vi "stop.vi"(3 "error in (no error)":errorcluster, 4 "stop":bool, 5 "A66xxSupply in":refnum<class "A66xxSupply.lvclass">) -> (0 "error out":errorcluster, 1 "Stopped":bool, 2 "A66xxSupply out":refnum<class "A66xxSupply.lvclass">)   [LabVIEW 2011, in "Hardware.lvlib" / "Channels.lvlib" / "A66xxSupply.lvclass"]
doc: "Abstract Method.\n\nStops the analog output. This vi indicates of the analog output has stopped, and can be used to actively stop the output."
uses:
  A66xxSupply.lvclass
  AnalogOutput.lvclass
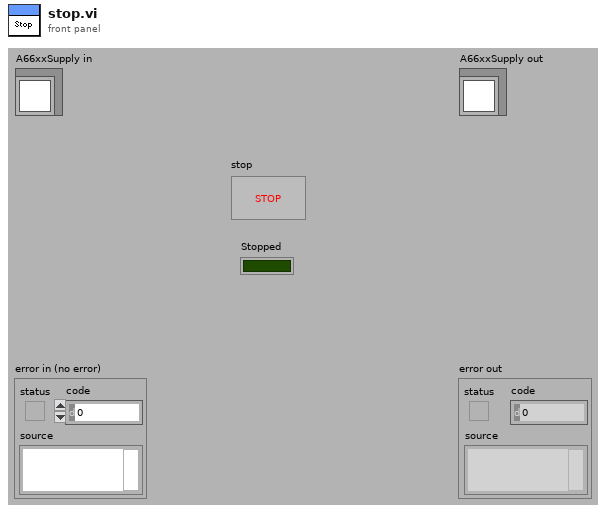
[diagram p1: front panel]
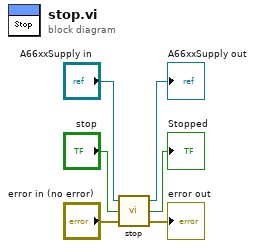
[diagram p0: block diagram]
diagram:
  n1 = call-parent "stop.vi"("error in (no error)"="error in (no error)", "stop"="stop", "AnalogOutput in"="A66xxSupply in") -> ("error out"=→"error out":errorcluster, "Stopped"=→"Stopped":bool, "AnalogOutput out"=→"A66xxSupply out":refnum<class "A66xxSupply.lvclass">)
